vi "02TRM800_NextCommand.vi"(8 "error in (no error)":errorcluster, 9 "Numeric":u32, 11 "Command":T1(ring)) -> (0 "error out":errorcluster, 3 "String":string)   [LabVIEW 2020]
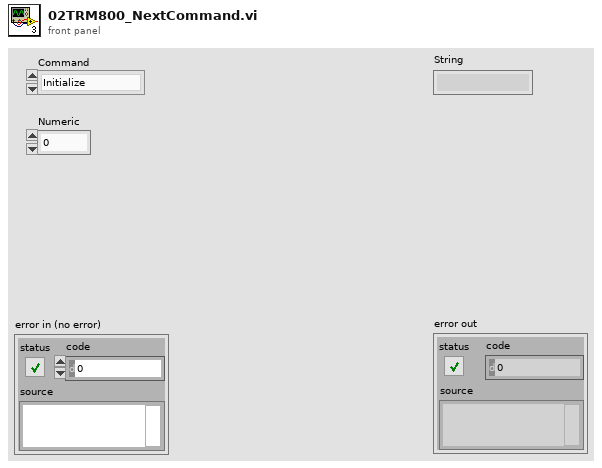
[diagram p1: front panel]
types:
  T1 = enum16{"Initialize", "Get", "SetInitCommands", "SetMPH", "SetInc"}
  T2 = cluster{"Command":enum16{"mph", "incq", "amps", "vin", "iamp", "vbus", "mtmp", "ptmp", "led1", "xmph", "cnfg", "inc", "led2", "part", "ver", "type", "loop", "err"}, "Parameter":string}
  T3 = enum16{"mph", "incq", "amps", "vin", "iamp", "vbus", "mtmp", "ptmp", "led1", "xmph", "cnfg", "inc", "led2", "part", "ver", "type", "loop", "err"}
  T4 = cluster{"Command":enum16{"mph", "incq", "amps", "vin", "iamp", "vbus", "mtmp", "ptmp", "led1", "xmph", "cnfg", "inc", "led2", "part", "ver", "type", "loop", "err"}, "Parameter":string}[]
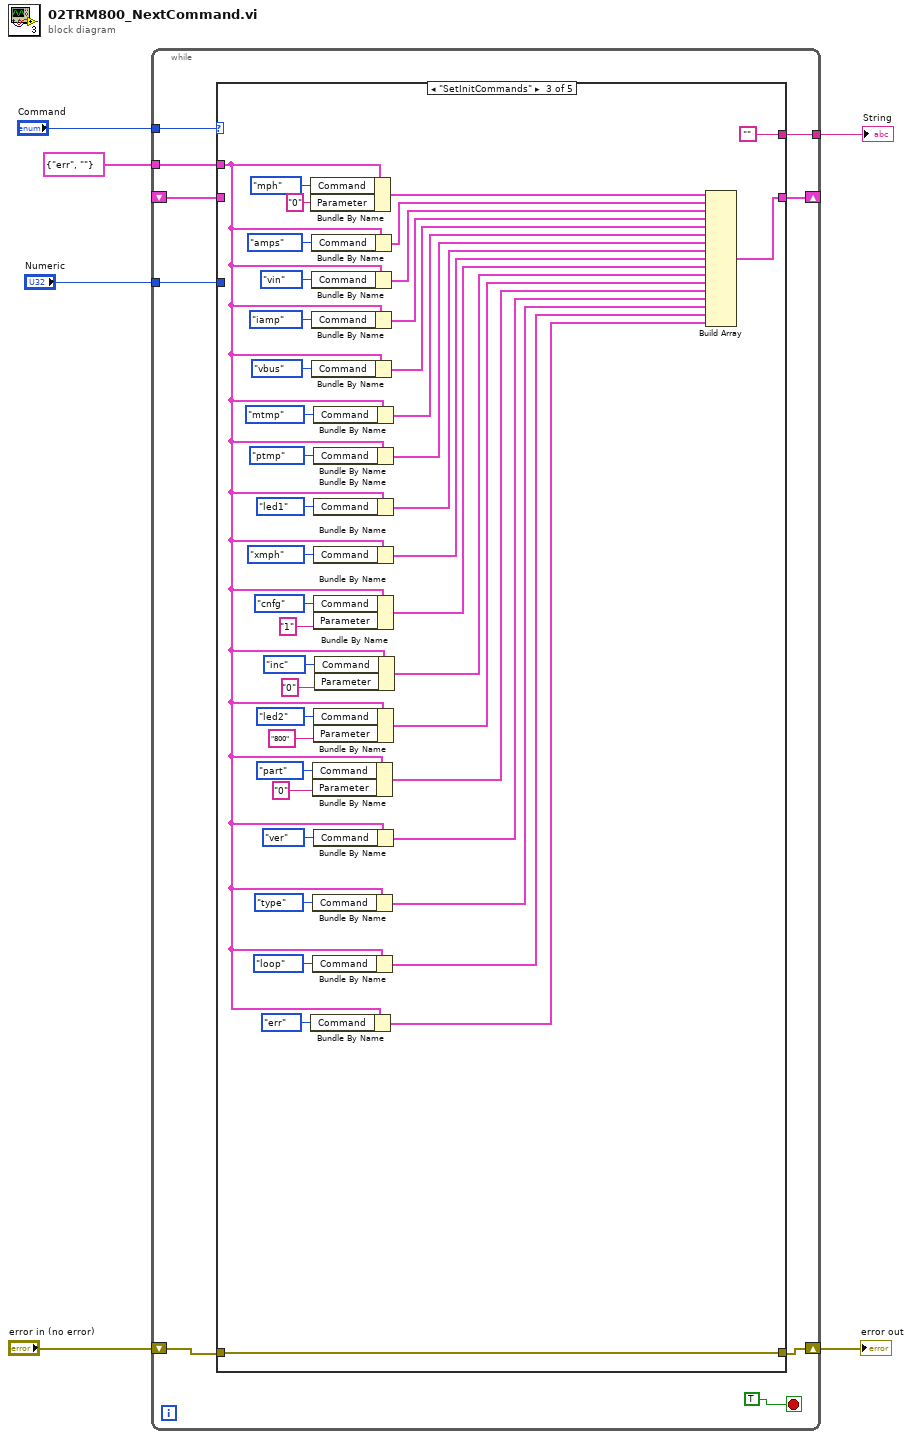
[diagram p0: block diagram]
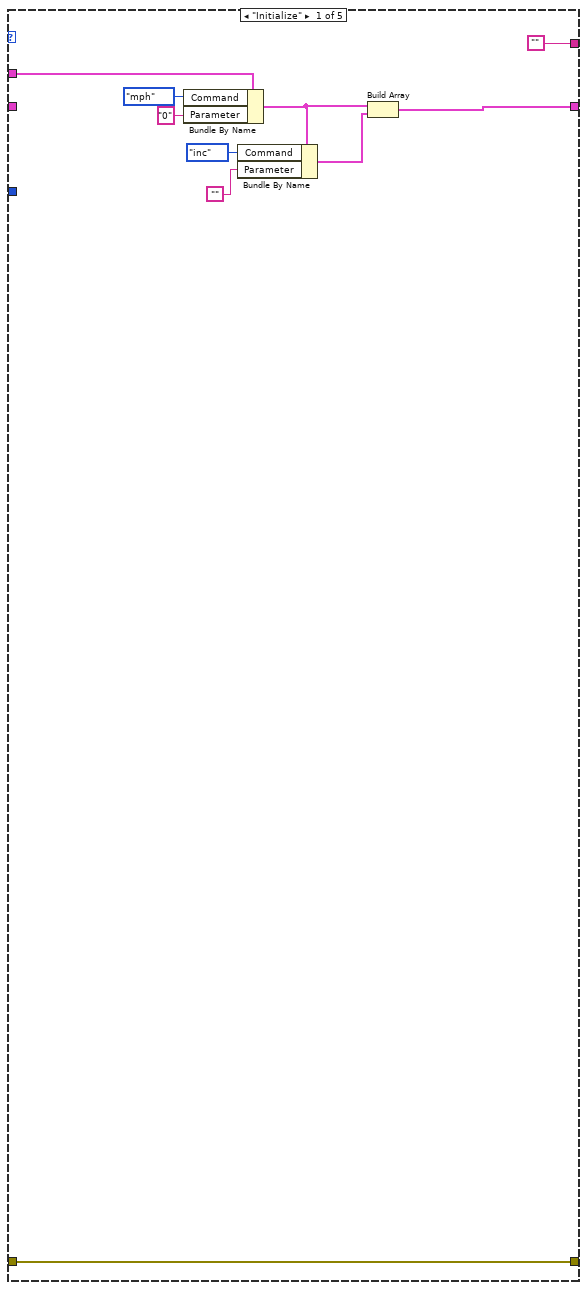
[diagram p2: hidden frame]
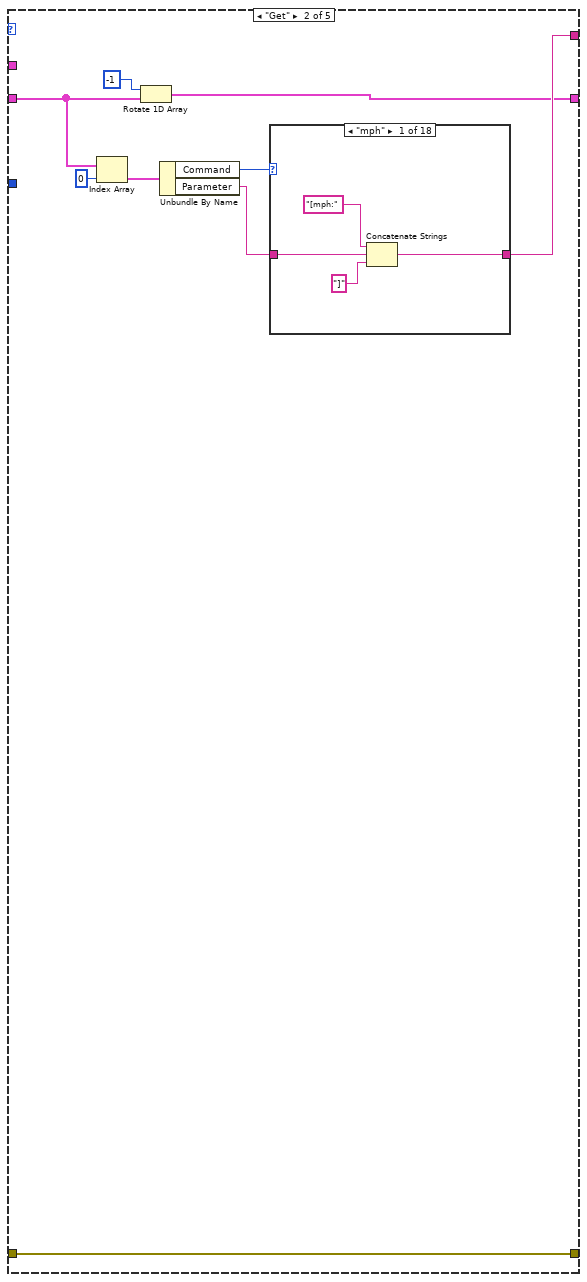
[diagram p3: hidden frame]
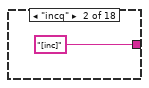
[diagram p4: hidden frame]
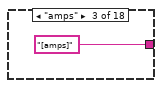
[diagram p5: hidden frame]
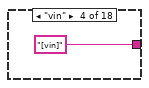
[diagram p6: hidden frame]
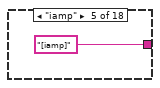
[diagram p7: hidden frame]
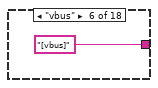
[diagram p8: hidden frame]
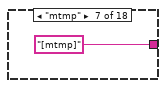
[diagram p9: hidden frame]
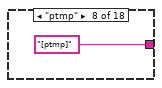
[diagram p10: hidden frame]
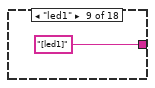
[diagram p11: hidden frame]
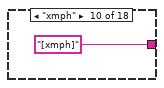
[diagram p12: hidden frame]
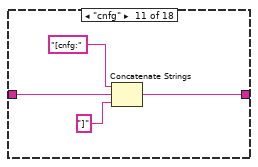
[diagram p13: hidden frame]
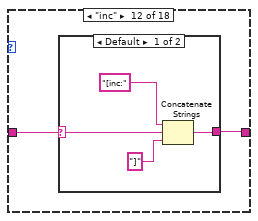
[diagram p14: hidden frame]
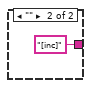
[diagram p15: hidden frame]
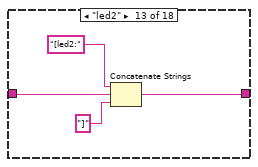
[diagram p16: hidden frame]
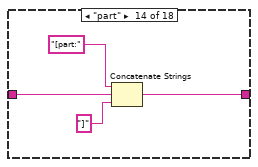
[diagram p17: hidden frame]
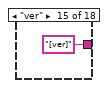
[diagram p18: hidden frame]
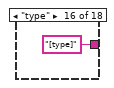
[diagram p19: hidden frame]
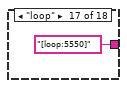
[diagram p20: hidden frame]
diagram:
  n1 = while {
    shift-right: [w12] -> w5
    shift-left: "error in (no error)" -> [w14]
    tunnel: "Command" -> [w15]
    tunnel: [w11] -> w3
    tunnel: T2 {"Command"=enum."err", "Parameter"=""} -> [w10]
    shift-right: [w9] -> _
    shift-left: _ -> [w8]
    tunnel: "Numeric" -> [w7]
    stop <- TRUE stop-if-true
    n2 = case shown="\"SetInitCommands\"" w15 {
      tunnel: w14 -> [w25 w34 w112 w118 w132]
      tunnel: [w25 w34 w112 w118 w132] -> w12
      tunnel: ["" w29 "" "" ""] -> w11
      tunnel: w10 -> [w24 _ w93 _ _]
      tunnel: [w22 w27 w88 w114 w128] -> w9
      tunnel: w8 -> [_ w28 _ w117 w131]
      tunnel: w7 -> [_ _ _ w116 w130]
      frame "Initialize" {
        n3 = Bundle By Name(cluster=w24, "Command"=T3."mph", "Parameter"="0") -> (w20:T2)
        n4 = Bundle By Name(cluster=w20, "Command"=T3."inc", "Parameter"="") -> (w19:T2)
        n5 = Build Array(w20, w19) -> (w22:T4)
      }
      frame "Get" {
        n6 = Index Array(array=w28, index=0) -> (element=w32:T2)
        n7 = Rotate 1D Array(1:w28, 2:-1 ("n")) -> (0:w27:T4)
        n8 = Unbundle By Name(w32) -> ("Command"=w31:T3, "Parameter"=w30:string)
        n9 = case shown="\"mph\"" w31 {
          tunnel: w30 -> [w38 _ _ _ _ _ _ _ _ _ w49 w53 w60 w64 _ _ _ _]
          tunnel: [w35 "[inc]" "[amps]" "[vin]" "[iamp]" "[vbus]" "[mtmp]" "[ptmp]" "[led1]" "[xmph]" w48 w52 w59 w63 "[ver]" "[type]" "[loop:5550]" "[err]"] -> w29
          frame "mph" {
            n10 = Concatenate Strings("[mph:", w38, "]" ("string")) -> (w35:string)
          }
          frame "incq" {
          }
          frame "amps" {
          }
          frame "vin" {
          }
          frame "iamp" {
          }
          frame "vbus" {
          }
          frame "mtmp" {
          }
          frame "ptmp" {
          }
          frame "led1" {
          }
          frame "xmph" {
          }
          frame "cnfg" {
            n11 = Concatenate Strings("[cnfg:", w49, "]" ("string")) -> (w48:string)
          }
          frame "inc" {
            n12 = case shown="Default" w53 {
              selector: w53 -> [w55 _]
              tunnel: [w54 "[inc]"] -> w52
              frame Default {
                n13 = Concatenate Strings("[inc:", w55, "]" ("string")) -> (w54:string)
              }
              frame "" {
              }
            }
          }
          frame "led2" {
            n14 = Concatenate Strings("[led2:", w60, "]" ("string")) -> (w59:string)
          }
          frame "part" {
            n15 = Concatenate Strings("[part:", w64, "]" ("string")) -> (w63:string)
          }
          frame "ver" {
          }
          frame "type" {
          }
          frame "loop" {
          }
          frame "err" {
          }
        }
      }
      frame "SetInitCommands" {
        n16 = Bundle By Name(cluster=w93, "Command"=T3."mph", "Parameter"="0") -> (w89:T2)
        n17 = Bundle By Name(cluster=w93, "Command"=T3."err") -> (w73:T2)
        n18 = Bundle By Name(cluster=w93, "Command"=T3."amps") -> (w87:T2)
        n19 = Bundle By Name(cluster=w93, "Command"=T3."vin") -> (w86:T2)
        n20 = Bundle By Name(cluster=w93, "Command"=T3."iamp") -> (w85:T2)
        n21 = Bundle By Name(cluster=w93, "Command"=T3."vbus") -> (w84:T2)
        n22 = Bundle By Name(cluster=w93, "Command"=T3."part", "Parameter"="0") -> (w71:T2)
        n23 = Bundle By Name(cluster=w93, "Command"=T3."type") -> (w75:T2)
        n24 = Bundle By Name(cluster=w93, "Command"=T3."loop") -> (w74:T2)
        n25 = Bundle By Name(cluster=w93, "Command"=T3."mtmp") -> (w83:T2)
        n26 = Bundle By Name(cluster=w93, "Command"=T3."ptmp") -> (w82:T2)
        n27 = Bundle By Name(cluster=w93, "Command"=T3."led1") -> (w81:T2)
        n28 = Bundle By Name(cluster=w93, "Command"=T3."xmph") -> (w80:T2)
        n29 = Bundle By Name(cluster=w93, "Command"=T3."cnfg", "Parameter"="1") -> (w79:T2)
        n30 = Bundle By Name(cluster=w93, "Command"=T3."led2", "Parameter"="800") -> (w77:T2)
        n31 = Bundle By Name(cluster=w93, "Command"=T3."ver") -> (w76:T2)
        n32 = Bundle By Name(cluster=w93, "Command"=T3."inc", "Parameter"="0") -> (w78:T2)
        n33 = Build Array(w89, w87, w86, w85, w84, w83, w82, w81, w80, w79, w78, w77, w71, w76, w75, w74, w73) -> (w88:T4)
      }
      frame "SetMPH" {
        n34 = Number To Hexadecimal String(2:w116) -> (0:w115:string)  [unwired: 1 in]
        n35 = for {
          tunnel: w117 -> [w121] mode=indexing
          tunnel: w115 -> [w120]
          tunnel: [w122] -> w114 mode=indexing
          n36 = Unbundle By Name(w121) -> ("Command"=w123:T3)
          n37 = case shown="\"mph\"" w123 {
            tunnel: [w125 w127] -> w122
            tunnel: w121 -> [w126 w127]
            tunnel: w120 -> [w124 _]
            frame "mph" {
              n38 = Bundle By Name(cluster=w126, "Parameter"=w124) -> (w125:T2)
            }
            frame Default {
            }
          }
        }
      }
      frame "SetInc" {
        n39 = Number To Hexadecimal String(2:w130) -> (0:w129:string)  [unwired: 1 in]
        n40 = for {
          tunnel: w131 -> [w135] mode=indexing
          tunnel: w129 -> [w134]
          tunnel: [w136] -> w128 mode=indexing
          n41 = Unbundle By Name(w135) -> ("Command"=w137:T3)
          n42 = case shown="\"inc\"" w137 {
            tunnel: [w139 w141] -> w136
            tunnel: w135 -> [w140 w141]
            tunnel: w134 -> [w138 _]
            frame "inc" {
              n43 = Bundle By Name(cluster=w140, "Parameter"=w138) -> (w139:T2)
            }
            frame Default {
            }
          }
        }
      }
    }
  }
  "error out" <- w5
  "String" <- w3
